vi "test Copy mixed integer cluster array.vi"(8 "error in (no error)":errorcluster, 11 "TestCase in":refnum<class "Malleable Tests.lvclass">) -> (0 "error out":errorcluster, 3 "TestCase out":refnum<class "Malleable Tests.lvclass">)   [LabVIEW 2020, in "Memory Manager Tests.lvlib" / "Malleable Tests.lvclass"]
uses:
  Malleable Tests.lvclass
  Malleable Type Tests/Malleable Type Tests.lvclass
  C:/dev/illuminated-g/LabVIEW-Memory/Source/Classes/Pointer/Pointer.lvclass
  f3b27a50-7d59-49d5-b9c9-ccb1b75a8e01.vi
  f3b27a50-7d59-49d5-b9c9-ccb1b75a8e01.vi/48144062-09e8-44d7-a914-3b058f1e4a5b.vi
  Source/Classes/Pointer/Write U64.vi
  Source/Classes/Pointer/Write U32.vi
  Source/Classes/Pointer/Write U16.vi
  Source/Classes/Pointer/Check Null Pointer.vi
  Source/Classes/Pointer/Get Size.vi
  Source/Classes/Pointer/Get Address.vi
  Source/Classes/Pointer/Errors.vi
  Source/Classes/Pointer/Out of Bounds.vi
  <vilib>/addons/_JKI Toolkits/VI Tester/TestCase.llb/TestCase.lvclass
  Source/Classes/Pointer/Pointer.lvclass
  C:/dev/illuminated-g/LabVIEW-Memory/Tests/Memory Manager/Malleable Type Tests/Malleable Type Tests.lvclass
  C:/Program Files (x86)/National Instruments/LabVIEW 2020/vi.lib/addons/_JKI Toolkits/VI Tester/TestCase.llb/TestCase.lvclass
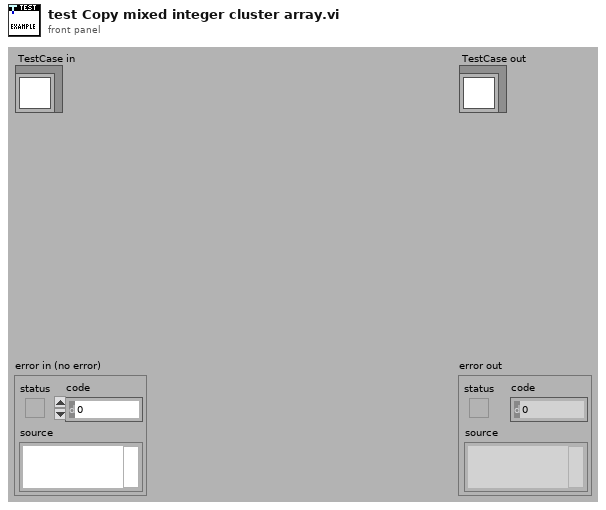
[diagram p1: front panel]
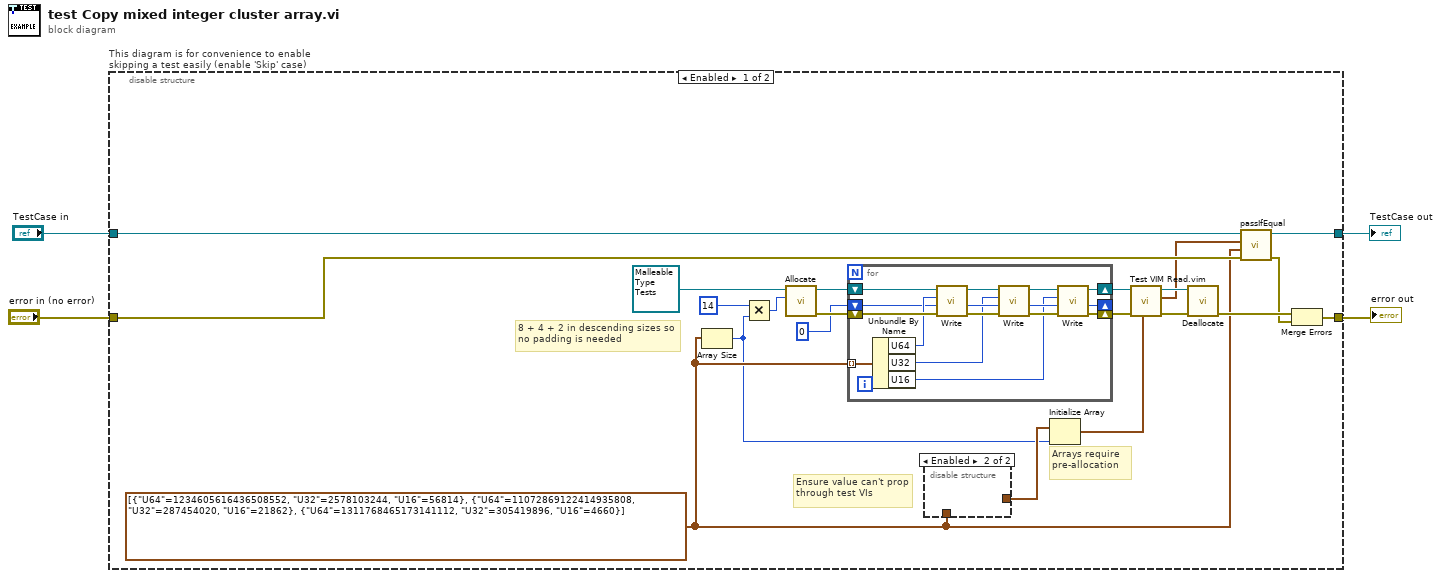
[diagram p0: block diagram]
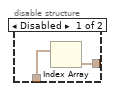
[diagram p2: hidden frame]
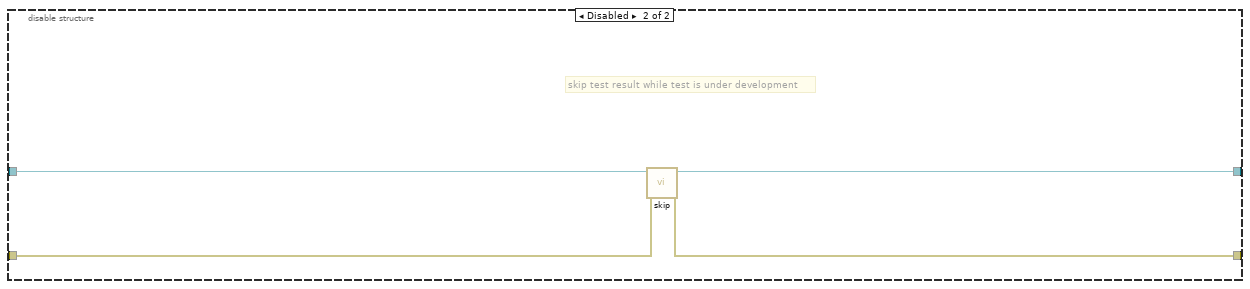
[diagram p3: hidden frame]
diagram:
  n1 = disable-structure "This diagram is for convenience to enable skipping a test easily (enable 'Skip' case)" shown="Enabled" {
    disable-tunnel: "TestCase in" -> [w12 w47]
    disable-tunnel: [w11 w45] -> w1
    disable-tunnel: [w10 w46] -> w3
    disable-tunnel: "error in (no error)" -> [w25 w44]
    frame Enabled {
      w8 = cluster{"U64":u64, "U32":u32, "U16":u16}[] [{"U64"=1234605616436508552, "U32"=2578103244, "U16"=56814}, {"U64"=11072869122414935808, "U32"=287454020, "U16"=21862}, {"U64"=1311768465173141112, "U32"=305419896, "U16"=4660}]
      # "Arrays require pre-allocation"
      # "Ensure value can't prop through test VIs"
      # "8 + 4 + 2 in descending sizes so no padding is needed"
      n2 = Array Size(array=w8) -> (size(s)=w5:i32)
      n3 = Multiply(x=u64 14 ("size"), y=w5) -> (x*y=w9:u64)
      n4 = call "Allocate.vi"("size"=w9, "Pointer type"=refnum<class "Malleable Type Tests.lvclass"> refnum ("Memory Manager Tests.lvlib:Malleable Type Tests.lvclass")) -> ("error out"=w21:errorcluster, "Pointer out"=w22:refnum<class "Malleable Type Tests.lvclass">)  [unwired: 8 in]
      n5 = for {
        shift-right: [w30] -> w20
        shift-left: w22 -> [w41]
        shift-right: [w29] -> w19
        shift-left: w21 -> [w40]
        tunnel: w8 -> [w28] mode=indexing
        shift-right: [w27] -> _
        shift-left: u64 0 ("offset + size") -> [w26]
        n6 = Unbundle By Name(w28) -> ("U64"=w39:u64, "U32"=w35:u32, "U16"=w31:u16)
        n7 = call-poly "Write.vi"("error in (no error)"=w40, "offset (0)"=w26, "value"=w39, "Pointer in"=w41) -> ("error out"=w37:errorcluster, "offset + size"=w36:u64, "Pointer out"=w38:refnum<class "Malleable Type Tests.lvclass">)  [unwired: 4 in, 1 out]
        n8 = call-poly "Write.vi"("error in (no error)"=w37, "offset (0)"=w36, "value"=w35, "Pointer in"=w38) -> ("error out"=w33:errorcluster, "offset + size"=w32:u64, "Pointer out"=w34:refnum<class "Malleable Type Tests.lvclass">)  [unwired: 4 in, 1 out]
        n9 = call-poly "Write.vi"("error in (no error)"=w33, "offset (0)"=w32, "value"=w31, "Pointer in"=w34) -> ("error out"=w29:errorcluster, "offset + size"=w27:u64, "Pointer out"=w30:refnum<class "Malleable Type Tests.lvclass">)  [unwired: 4 in, 1 out]
      }
      n10 = disable-structure shown="Enabled" {
        disable-tunnel: w8 -> [w43 _]
        disable-tunnel: [w42 _] -> w18
        frame Disabled {
          n11 = Index Array(array=w43) -> (element=w42:cluster{"U64":u64, "U32":u32, "U16":u16})  [unwired: 1 in]
        }
        frame Enabled {
        }
      }
      n12 = Initialize Array(w18, w5) -> (w6:cluster{"U64":u64, "U32":u32, "U16":u16}[])
      n13 = call "Test VIM Read.vim"("Type"=w6, "error in (no error)"=w19, "Malleable Type Tests in"=w20) -> ("error out"=w17:errorcluster, "Value"=w14:cluster{"U64":u64, "U32":u32, "U16":u16}[], "Malleable Type Tests out"=w16:refnum<class "Malleable Type Tests.lvclass">)  [unwired: 6 in]
      n14 = call "Deallocate.vi"("error in (no error)"=w17, "Pointer"=w16) -> ("error out"=w15:errorcluster)  [unwired: 8 in, 1 out]
      n15 = call-dynamic "passIfEqual.vi"("error in (no error)"=w25, "y"=w8, "x"=w14, "TestCase in"=w12) -> ("error out"=w13:errorcluster, "TestCase out"=w11:refnum<class "Malleable Tests.lvclass">)  [unwired: 6 in]
      n16 = Merge Errors(w15, w13) -> (w10:errorcluster)
    }
    frame Disabled {
      # "skip test result while test is under development"
      n17 = call <vilib>:"skip.vi"("error in (no error)"=w44, "TestCase in"=w47) -> ("error out"=w46:errorcluster, "TestCase out"=w45:refnum<class "Malleable Tests.lvclass">)  [unwired: 8 in]
    }
  }
  "error out" <- w3
  "TestCase out" <- w1
